vi "DriveSetGyroZero.vi"(11 "GyroZero":dbl) -> ()   [LabVIEW 2020]
doc: "Set GyroZero\n\nInputs:\n--GyroZero--Double--set gyro zero"
uses:
  DriveGlobal.vi
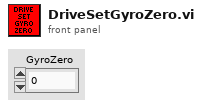
[diagram p1: front panel]
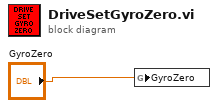
[diagram p0: block diagram]
diagram:
  n1 = global write "DriveGlobal.vi" "GyroZero"("GyroZero") -> ()
